vi "Auth Extra.vi"(8 "error in (no error)":errorcluster, 10 "authextra in":string="{}", 11 "TicketAuthentactor in":refnum<class "TicketAuthentactor.lvclass">) -> (0 "error out":errorcluster, 2 "authextra":string caption="authextra out", 3 "TicketAuthentactor out":refnum<class "TicketAuthentactor.lvclass">)   [LabVIEW 2020]
uses:
  TicketAuthentactor.lvclass
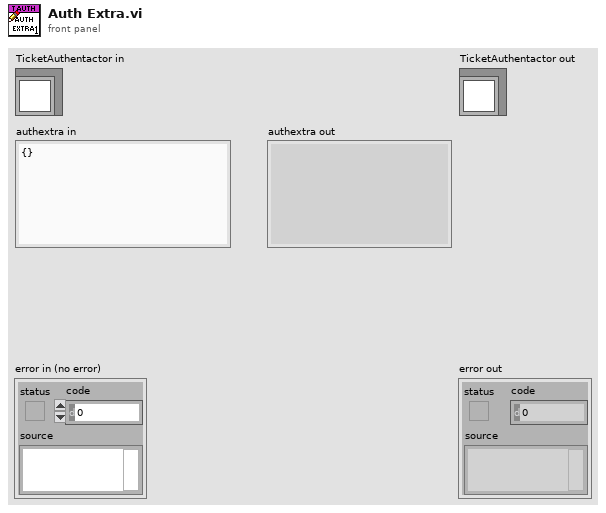
[diagram p1: front panel]
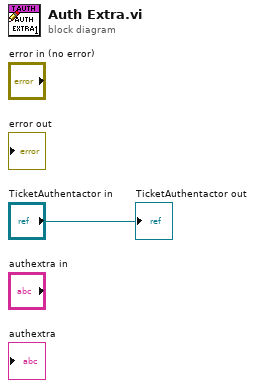
[diagram p0: block diagram]
diagram:
  "TicketAuthentactor out" <- "TicketAuthentactor in"
